vi "PING rising 1 time.vi"() -> ()   [LabVIEW 2019]
panel:
  out "overflow":bool
  in  "all time 1":u32
  in  "rising time 1":u32
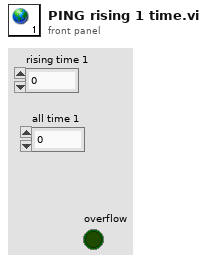
[diagram p1: front panel]
diagram:
